vi "Register Configuration and Results.vi"(8 "error in (no error)":errorcluster, 10 "Measurement":refnum<class "MeasurementPluginService.lvclass">, 11 "gRPC ID":T1) -> (0 "error out":errorcluster, 3 "gRPC ID Out":T1)   [LabVIEW 2020, in "MeasurementLink Measurement Server.lvlib"]
uses:
  MeasurementLink Measurement Server.lvlib
  <vilib>/gRPC/LabVIEW gRPC Library/grpc-lvsupport-release.lvlib
  Classes/MeasurementPluginService/MeasurementPluginService.lvclass
  <vilib>/gRPC/LabVIEW gRPC Library/Shared/grpcId.ctl
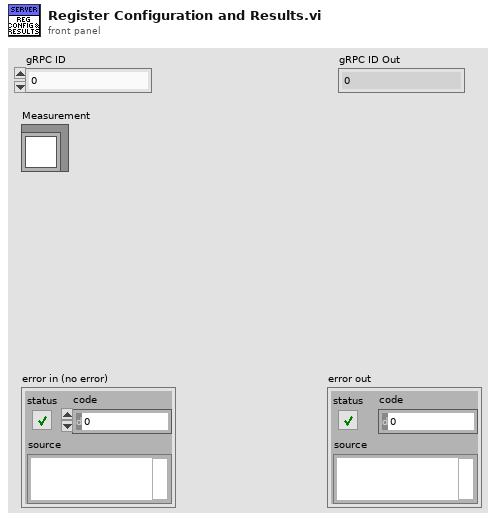
[diagram p1: front panel]
types:
  T1 = typedef "grpc-lvsupport-release.lvlib/grpcId.ctl" = u64
  T2 = typedef "MeasurementLink Measurement Server.lvlib/MeasurementPluginService.lvclass/Plugin Paths.ctl" = cluster{"Get Measurement Details VI Path":path, "Get Type Specializations VI Path":path, "Get UI Details VI Path":path, "Measurement Logic VI Path":path, "Measurement Configuration CTL Path":path, "Measurement Results CTL Path":path}
  T3 = typedef "grpc-lvsupport-release.lvlib/Message Metadata.ctl" = cluster{"Version":i32, "Name":string, "Type Url":string, "Elements":T4[]}
  T4 = typedef "grpc-lvsupport-release.lvlib/Message Element Metadata.ctl" = cluster{"Embedded Message Name":string, "Protobuf Index":i32, "MessageElementType":T5, "Repeated":bool}
  T5 = typedef "grpc-lvsupport-release.lvlib/Message Element Type.ctl" = enum32{"Int32Value", "FloatValue", "DoubleValue", "BoolValue", "StringValue", "MessageValue", "Int64Value", "UInt32Value", "UInt64Value", "EnumValue", "Bytes", "Fixed64", "Fixed32", "SFixed64", "SFixed32", "SInt64", "SInt32"}
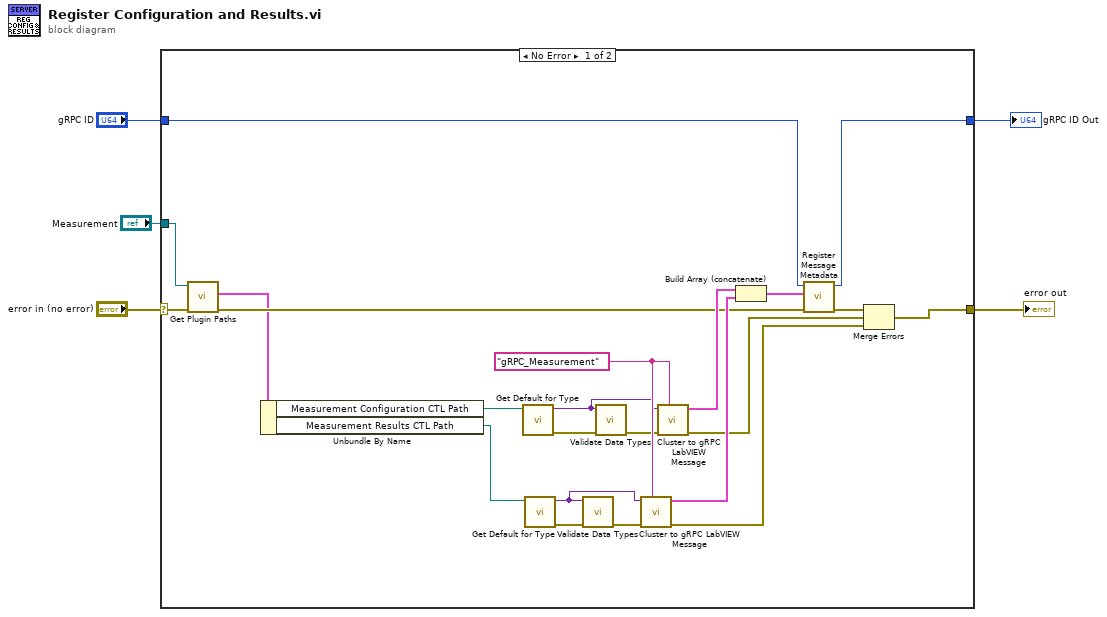
[diagram p0: block diagram]
diagram:
  n1 = case shown="No Error" "error in (no error)" {
    selector: "error in (no error)" -> [w16 w29]
    tunnel: [w20 w28] -> w2
    tunnel: [w23 w29] -> w5
    tunnel: "gRPC ID" -> [w19 w28]
    tunnel: "Measurement" -> [w17 _]
    frame No Error {
      w18 = "gRPC_Measurement" ("Package Name")
      n2 = call-dynamic "Get Plugin Paths.vi"("error in (no error)"=w16, "MeasurementService in"=w17) -> ("error out"=w15:errorcluster, "Plugin Paths"=w14:T2)  [unwired: 7 in, 1 out]
      n3 = Unbundle By Name(w14) -> ("Measurement Configuration CTL Path"=w13:path, "Measurement Results CTL Path"=w12:path)
      n4 = call "Get Default for Type.vi"("Path of Type"=w13) -> ("error out"=w11:errorcluster, "Default for Type"=w10:variant)  [unwired: 9 in]
      n5 = call "Get Default for Type.vi"("Path of Type"=w12) -> ("error out"=w8:errorcluster, "Default for Type"=w7:variant)  [unwired: 9 in]
      n6 = call "Validate Data Types.vi"("error in (no error)"=w8, "Cluster"=w7) -> ("error out"=w6:errorcluster)  [unwired: 9 in]
      n7 = call "Validate Data Types.vi"("error in (no error)"=w11, "Cluster"=w10) -> ("error out"=w9:errorcluster)  [unwired: 9 in]
      n8 = call <vilib>:"Cluster to gRPC LabVIEW Message.vi"("Package Name"=w18, "error in"=w6, "Cluster"=w7) -> ("error out"=w22:errorcluster, "gRPC Message Metadata []"=w25:T3[])  [unwired: 7 in]
      n9 = call <vilib>:"Cluster to gRPC LabVIEW Message.vi"("Package Name"=w18, "error in"=w9, "Cluster"=w10) -> ("error out"=w21:errorcluster, "gRPC Message Metadata []"=w26:T3[])  [unwired: 7 in]
      n10 = Build Array (concatenate)(w26, w25) -> (w24:T3[])
      n11 = call <vilib>:"Register Message Metadata.vi"("error in"=w15, "Messages"=w24, "gRPCid in"=w19) -> ("error out"=w27:errorcluster, "gRPCid out"=w20:T1)  [unwired: 7 in]
      n12 = Merge Errors(w27, w21, w22) -> (w23:errorcluster)
    }
    frame Error {
    }
  }
  "error out" <- w5
  "gRPC ID Out" <- w2
